vi "Main_Init_App.vi"(8 "error in (no error)":errorcluster) -> (0 "error out":errorcluster, 2 "Main ini path":string="C:\\ProgramData\\Noffz\\mmW_Service\\mmw_Service.ini")   [LabVIEW 2019, in "Service.lvlib"]
uses:
  Service.lvlib
  <vilib>/Field R&D Services/Logger/Type Definitions/Severity.ctl
  <vilib>/Field R&D Services/Logger/Field_RnD_Services_Logger_Toolkit.lvlib
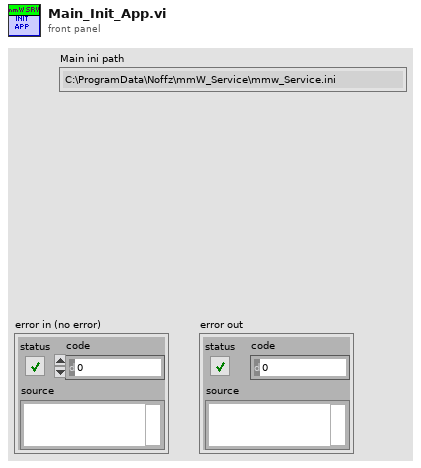
[diagram p1: front panel]
types:
  T1 = typedef "Field_RnD_Services_Logger_Toolkit.lvlib/Severity.ctl" = enum16{"Benign", "Warning", "Recoverable", "Fatal"}
  T2 = enum32{"invalid app kind", "Development System", "Run Time System", "Student Edition", "Embedded LabVIEW", "Evaluation", "Custom"}
  T3 = typedef "Service.lvlib/AppData.ctl" = cluster{"MsgQ":refnum<queue>, "Stop?":bool, "zmq sessions":cluster{"Control_endpoint":string, "Instr_endpoint":string}, "control-loop":cluster{"fromUI-Q":refnum<queue>, "toUI":refnum<user-event>, "Control_endpoint":string}, "UI-loop":cluster{"evnt_ref":refnum<event-registration>}, "logging":cluster{"level":dbl, "verbosity":dbl, "path":string, "Listener_ID":string}, "general_settings":cluster{"mmW_instr_ini_path":string, "mmW_instr_pid_path":string}}
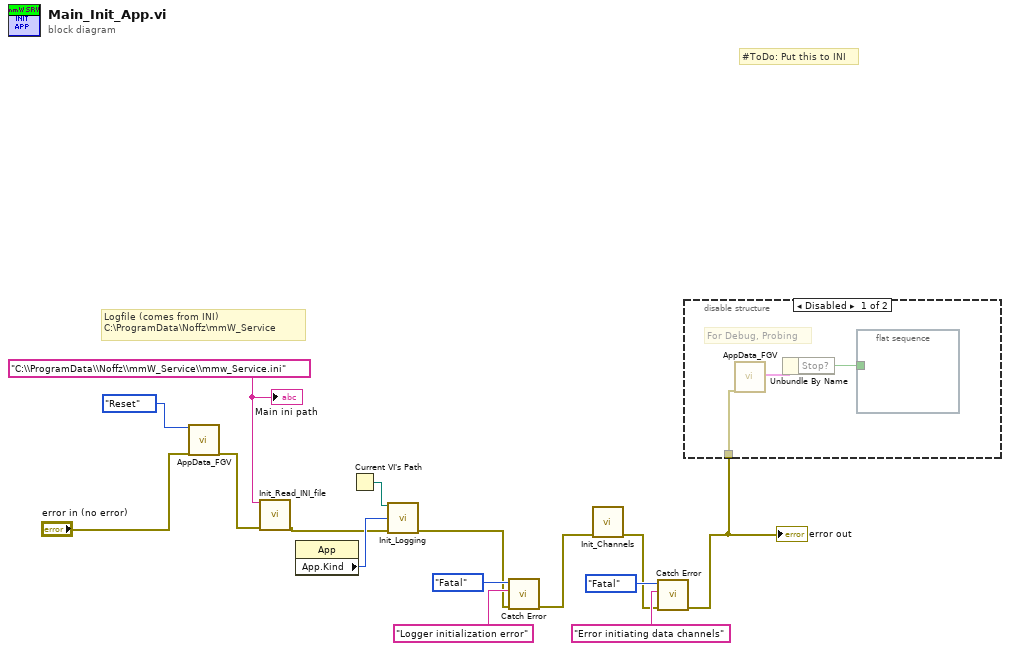
[diagram p0: block diagram]
diagram:
  w5 = "C:\\ProgramData\\Noffz\\mmW_Service\\mmw_Service.ini" ("Message")
  # "Logfile (comes from INI)\nC:\\ProgramData\\Noffz\\mmW_Service"
  # "#ToDo: Put this to INI"
  n1 = call "AppData_FGV.vi"("Mode"=enum16{"Get", "Set", "Reset"}."Reset", "error in (no error)"="error in (no error)") -> ("error out"=w7:errorcluster)  [unwired: 16 in, 1 out]
  n2 = call "Init_Read_INI_file.vi"("Path to INI"=w5, "error in (no error)"=w7) -> ("error out"=w6:errorcluster)  [unwired: 13 in]
  n3 = property class="App"() -> ("App.Kind"=w14:T2)  [unwired: 2 in, 2 out]
  n4 = Current VI's Path() -> (path=w9:path)
  n5 = call "Init_Logging.vi"("Main Init VI path"=w9, "App.Kind"=w14, "error in (no error)"=w6) -> ("error out"=w4:errorcluster)  [unwired: 12 in]
  n6 = call <vilib>:"Catch Error.vi"("Error In"=w4, "Source"="Logger initialization error", "Severity"=Severity."Fatal") -> ("Error Out"=w3:errorcluster)  [unwired: 8 in]
  n7 = call "Init_Channels.vi"("error in (no error)"=w3) -> ("error out"=w2:errorcluster)  [unwired: 14 in]
  n8 = call <vilib>:"Catch Error.vi"("Error In"=w2, "Source"="Error initiating data channels", "Severity"=Severity."Fatal") -> ("Error Out"=w1:errorcluster)  [unwired: 8 in]
  "error out" <- w1
  n9 = disable-structure shown="Disabled" {
    disable-tunnel: w1 -> [w18 _]
    frame Disabled {
      # "For Debug, Probing"
      n10 = call "AppData_FGV.vi"("error in (no error)"=w18) -> ("AppData out"=w17:T3)  [unwired: 17 in, 1 out]
      n11 = Unbundle By Name(w17) -> ("Stop?"=w16:bool)
      n12 = flat-sequence {
        tunnel: w16 -> [_]
        frame #0 {
        }
      }
    }
    frame Enabled {
    }
  }
  "Main ini path" <- w5
